vi "Open Arms.vi"(8 "error in (no error)":errorcluster, 11 "Grabber in":refnum<class "Grabber.lvclass">) -> (0 "error out":errorcluster, 3 "Grabber out":refnum<class "Grabber.lvclass">)   [LabVIEW 2014, in "Grabber.lvlib" / "Grabber.lvclass"]
uses:
  Grabber.lvclass
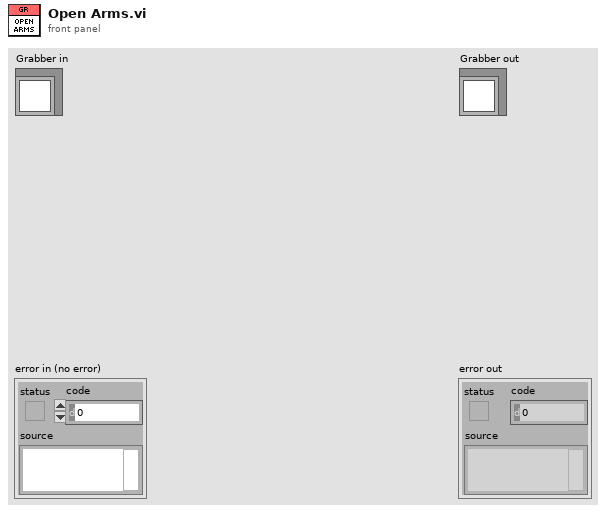
[diagram p1: front panel]
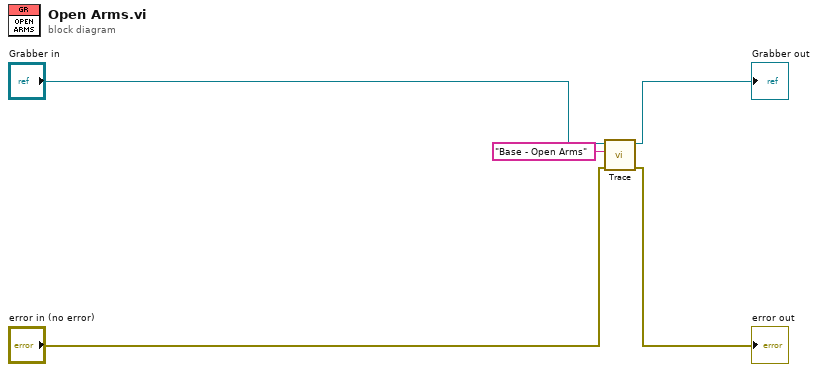
[diagram p0: block diagram]
diagram:
  n1 = call-dynamic "Trace.vi"("error in (no error)"="error in (no error)", "System Action"="Base - Open Arms", "System Actor in"="Grabber in") -> ("error out"=→"error out":errorcluster, "System Actor out"=→"Grabber out":refnum<class "Grabber.lvclass">)  [unwired: 7 in]
